vi "receive.vi"(8 "error in (no error)":errorcluster, 11 "Modbus in":refnum<class "Modbus.lvclass">) -> (0 "error out":errorcluster, 2 "Data":T1[](array[typedef]) {"Data" format="%02x"}, 3 "Modbus out":refnum<class "Modbus.lvclass">)   [LabVIEW 2015, in "Modbus.lvclass"]
uses:
  Modbus.lvclass
  Typedefs/Frame.ctl
  Modbus.lvclass/Modbus.ctl
  Typedefs/RTTypeDefs.lvlib
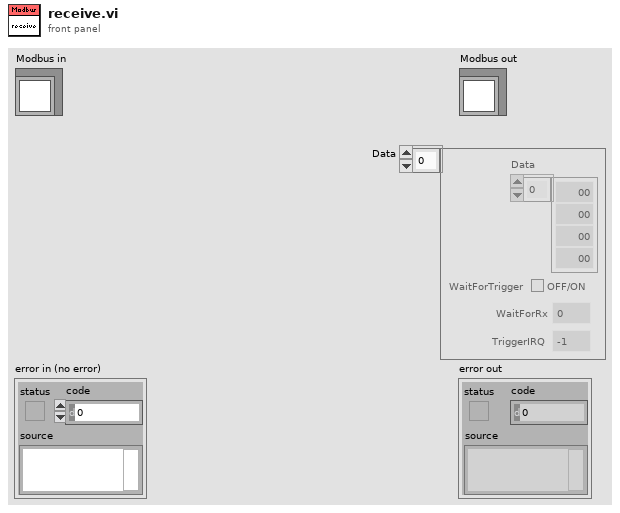
[diagram p1: front panel]
types:
  T1 = typedef "RTTypeDefs.lvlib/Frame.ctl" = cluster{"Data":u8[], "WaitForTrigger":bool, "WaitForRx":u16, "TriggerIRQ":i16}
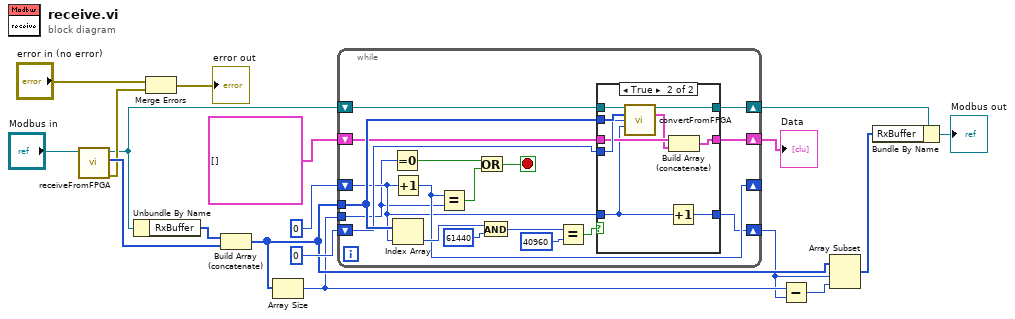
[diagram p0: block diagram]
diagram:
  n1 = call-dynamic "receiveFromFPGA.vi"("Modbus in"="Modbus in") -> ("error out"=w15:errorcluster, "Data"=w17:u16[], "Modbus out"=w10:refnum<class "Modbus.lvclass">)  [unwired: 8 in]
  n2 = Unbundle By Name(w10) -> ("RxBuffer"=w18:u16[])
  n3 = Merge Errors("error in (no error)", w15) -> (→"error out":errorcluster)
  n4 = Build Array (concatenate)(w18, w17) -> (w7:u16[])
  n5 = Array Size(array=w7) -> (size(s)=w6:i32)
  n6 = while {
    shift-right: [w31] -> _
    shift-left: 0 -> [w27]
    shift-right: [w26] -> w5
    shift-left: 0 -> [w28]
    tunnel: w7 -> [w29]
    tunnel: w6 -> [w22]
    shift-right: [w25] -> w8
    shift-left: w10 -> [w30]
    shift-right: [w23] -> w1
    shift-left: T1[] [] ("Data") -> [w24]
    stop <- w19 stop-if-true
    n7 = Equal To 0?(x=w22) -> (x = 0?=w21:bool)
    n8 = Increment(x=w27) -> (x+1=w31:i32)
    n9 = Index Array(array=w29, index=w27) -> (element=w36:u16)
    n10 = Equal?(x=w31, y=w22) -> (x = y?=w20:bool)
    n11 = Or(x=w21, y=w20) -> (x .or. y?=w19:bool)
    n12 = And(x=w36, y=u16 61440) -> (x .and. y?=w34:u16)
    n13 = Equal?(x=w34, y=u16 40960) -> (x = y?=w32:bool)
    n14 = case shown="True" w32 {
      tunnel: w30 -> [w38 w48]
      tunnel: w29 -> [_ w47]
      tunnel: w28 -> [w39 w46]
      tunnel: w27 -> [_ w41]
      tunnel: [w39 w40] -> w26
      tunnel: [w38 w45] -> w25
      tunnel: w24 -> [w37 w44]
      tunnel: [w37 w43] -> w23
      frame False {
      }
      frame True {
        n15 = call "convertFromFPGA.vi"("Modbus in"=w48, "Data"=w47, "StartIndex"=w46, "StopIndex"=w41) -> ("Modbus out"=w45:refnum<class "Modbus.lvclass">, "Frame"=w42:T1)  [unwired: 9 in, 1 out]
        n16 = Increment(x=w41) -> (x+1=w40:i32)
        n17 = Build Array (concatenate)(w44, w42) -> (w43:T1[])
      }
    }
  }
  "Data" <- w1
  n18 = Subtract(x=w6, y=w5) -> (x-y=w4:i32)
  n19 = Array Subset(array=w7, index=w5, length=w4) -> (w3:u16[])
  n20 = Bundle By Name(cluster=w8, "RxBuffer"=w3) -> (→"Modbus out":refnum<class "Modbus.lvclass">)
